vi "SE FP hindbrain ACT.vi"(4 "MSpeed":dbl(slide) scale=0.0005..0.0025 scale format="%#.1g", 6 "Manual?":bool=TRUE, 7 "GPS?":bool=TRUE, 8 "error in":errorcluster, 9 "Act Com":T1, 10 "MHeading":dbl(slide) scale=0.0005..0.0025 scale format="%_1f", 11 "Current Boat Speed":dbl) -> (0 "error out":errorcluster, 1 "Speed":dbl min=-9.0 max=9.0 step=1.0, 2 "Desired \nRudder":dbl, 3 "Desired\nSpeed":dbl, 5 "Rudder":dbl min=-45.0 max=45.0 step=1.0)   [LabVIEW 2014]
doc: "This vi has two functions: it selects between manual and auto mode and it converts the incoming value into speed and rudder control values."
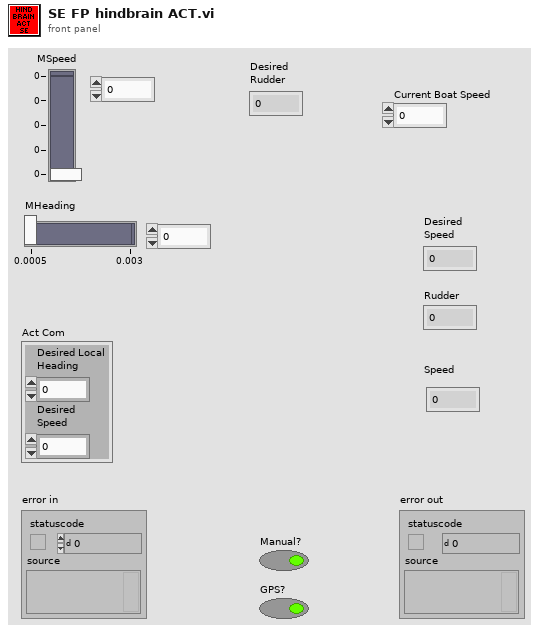
[diagram p1: front panel]
types:
  T1 = cluster{"Desired Local\nHeading":dbl, "Desired\nSpeed":dbl}
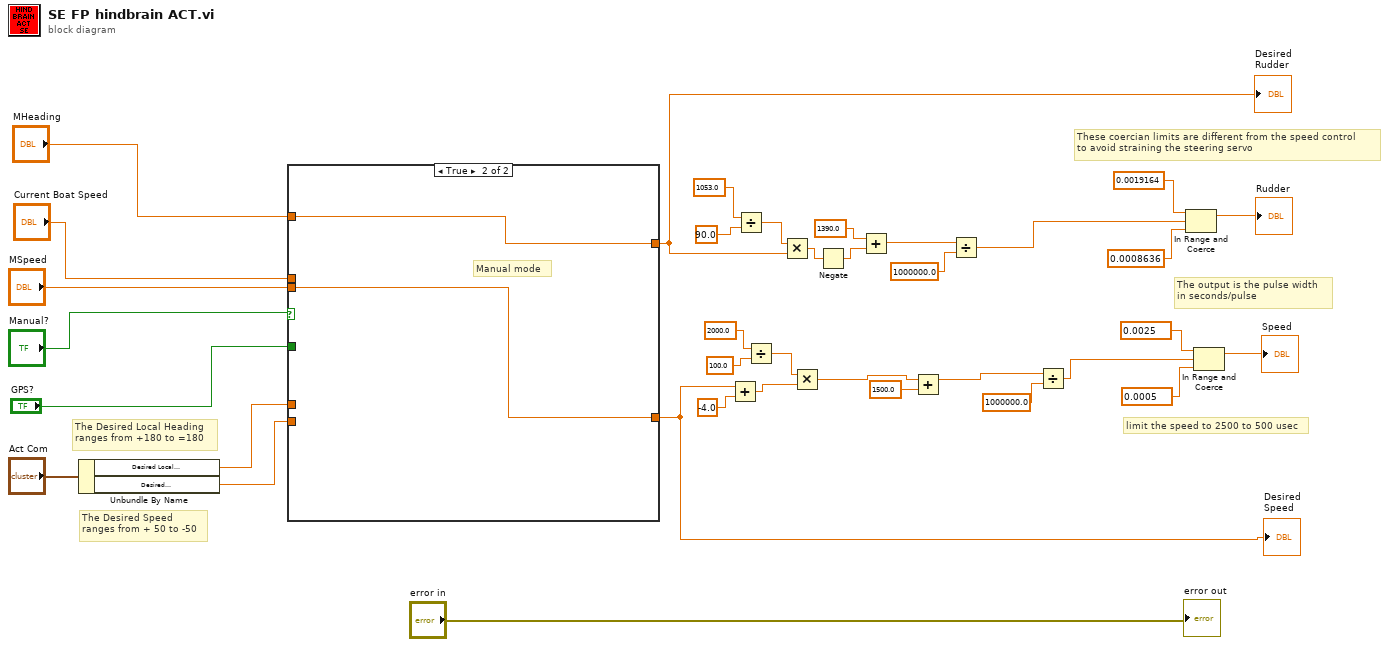
[diagram p0: block diagram]
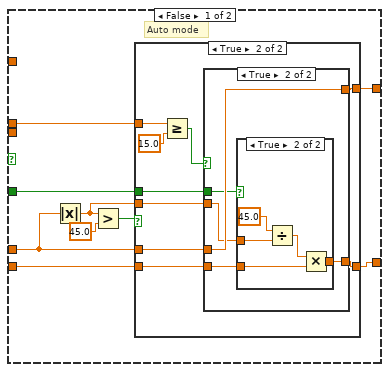
[diagram p2: hidden frame]
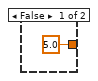
[diagram p5: hidden frame]
diagram:
  # "These coercian limits are different from the speed control\nto avoid straining the steering servo"
  # "The output is the pulse width\nin seconds/pulse"
  # "The Desired Local Heading\nranges from +180 to =180"
  # "The Desired Speed\nranges from + 50 to -50"
  # "limit the speed to 2500 to 500 usec"
  n1 = Unbundle By Name("Act Com") -> ("Desired Local\nHeading"=w28:dbl, "Desired\nSpeed"=w27:dbl)
  n2 = case shown="True" "Manual?" {
    tunnel: w28 -> [w39 _]
    tunnel: [w42 w71] -> w1
    tunnel: w27 -> [w41 _]
    tunnel: [w40 w70] -> w4
    tunnel: "MHeading" -> [_ w71]
    tunnel: "MSpeed" -> [_ w70]
    tunnel: "Current Boat Speed" -> [w43 _]
    tunnel: "GPS?" -> [w37 _]
    frame False {
      # "Auto mode"
      n3 = Absolute Value(x=w39) -> (abs(x)=w38:dbl)
      n4 = Greater?(x=w38, y=45.0 ("x")) -> (0:w44:bool)
      n5 = case shown="True" w44 {
        tunnel: w43 -> [_ w56]
        tunnel: [w46 w51] -> w42
        tunnel: w41 -> [w47 w52]
        tunnel: [w47 w53] -> w40
        tunnel: w39 -> [w46 w50]
        tunnel: w38 -> [_ w49]
        tunnel: w37 -> [_ w48]
        frame False {
        }
        frame True {
          n6 = Greater Or Equal?(x=w56, y=15.0) -> (x >= y?=w54:bool)
          n7 = case shown="True" w54 {
            tunnel: [w58 w63] -> w53
            tunnel: w52 -> [w58 w60]
            tunnel: [w57 w62] -> w51
            tunnel: w50 -> [w57 w62]
            tunnel: w49 -> [_ w61]
            tunnel: w48 -> [_ w59]
            frame False {
            }
            frame True {
              n8 = case shown="True" w59 {
                tunnel: [5.0 w69] -> w63
                tunnel: w61 -> [_ w68]
                tunnel: w60 -> [_ w67]
                frame False {
                }
                frame True {
                  n9 = Divide(x=45.0, y=w68) -> (x/y=w66:dbl)
                  n10 = Multiply(x=w66, y=w67) -> (x*y=w69:dbl)
                }
              }
            }
          }
        }
      }
    }
    frame True {
      # "Manual mode"
    }
  }
  "Desired \nRudder" <- w1
  "Desired\nSpeed" <- w4
  n11 = Add(x=w4, y=-4.0) -> (x+y=w9:dbl)
  n12 = Divide(x=1053.0, y=90.0) -> (x/y=w21:dbl)
  n13 = Divide(x=2000.0, y=100.0) -> (x/y=w17:dbl)
  n14 = Multiply(x=w21, y=w1) -> (x*y=w6:dbl)
  n15 = Multiply(x=w17, y=w9) -> (x*y=w8:dbl)
  n16 = Negate(x=w6) -> (-x=w5:dbl)
  n17 = Add(x=1390.0, y=w5) -> (x+y=w15:dbl)
  n18 = Add(x=w8, y=1500.0) -> (x+y=w14:dbl)
  n19 = Divide(x=w15, y=1000000.0) -> (x/y=w2:dbl)
  n20 = Divide(x=w14, y=1000000.0) -> (x/y=w3:dbl)
  n21 = In Range and Coerce(upper limit=0.0019164 ("t"), x=w2, lower limit=0.0008636 ("t")) -> (coerced(x)=→"Rudder":dbl)  [unwired: 1 out]
  n22 = In Range and Coerce(upper limit=0.0025 ("t"), x=w3, lower limit=0.0005 ("t")) -> (coerced(x)=→"Speed":dbl)  [unwired: 1 out]
  "error out" <- "error in"
